vi "getAO.vi"(8 "error in (no error)":errorcluster, 11 "Instrument.LockinAPI in":refnum<class "Instrument.LockinAPI.lvclass">) -> (0 "error out":errorcluster, 2 "AOconfig":T1[](array[typedef]), 3 "Instrument.LockinAPI out":refnum<class "Instrument.LockinAPI.lvclass">)   [LabVIEW 2019, in "Instrument.LockinAPI.lvclass"]
doc: "API to get the results of lockin calculation.\n\nIf address=\"\", this API reads from localhost\nIf address is remote lockin, you need to add this computer to allowed whitelist on the lockin computer you are trying to access."
uses:
  Instrument.LockinAPI.lvclass
  C:/Users/patrick/Documents/GitHub/Instrument-Framework/lvsrc/Instrument/Instrument.lvclass
  Typedefs/LockinAPI.AOconfig--Cluster.ctl
  Typedefs/LockinAPI.Commands--Enum.ctl
  8040a651-251f-490b-970e-b747a6a9edfe.vi
  8040a651-251f-490b-970e-b747a6a9edfe.vi/73a72ad9-01cb-4234-818c-ca637e3ba3a8.vi
  8040a651-251f-490b-970e-b747a6a9edfe.vi/73a72ad9-01cb-4234-818c-ca637e3ba3a8.vi/1562ab7a-2f08-4fb7-b07f-5ee483217534.vi
  8040a651-251f-490b-970e-b747a6a9edfe.vi/73a72ad9-01cb-4234-818c-ca637e3ba3a8.vi/22dc2966-521d-4730-be92-c328b528c3eb.vi
  Instrument/Protected/Validate API method.vi
  Instrument/Private/Get RC Connection Status.vi
  Instrument/API/Send and Receive.vi
  <vilib>/Utility/Data Type/Get Type Information.vi
  <vilib>/JDP Science/JSONtext/JSON text to Variant.vi
  <vilib>/JDP Science/JSONtext/LVClass Serializer/JSONtext LVClass Serializer.lvclass
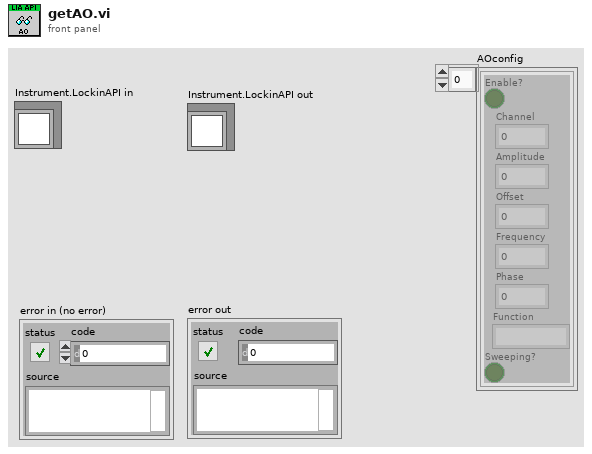
[diagram p1: front panel]
types:
  T1 = typedef "Instrument.LockinAPI.lvclass/LockinAPI.AOconfig--Cluster.ctl" = cluster{"Enable?":bool, "Channel":i32, "Amplitude":dbl, "Offset":dbl, "Frequency":dbl, "Phase":dbl, "Function":string, "Sweeping?":bool}
  T2 = typedef "Instrument.LockinAPI.lvclass/LockinAPI.Commands--Enum.ctl" = enum16{"setAI", "setAO", "setAO_Amplitude", "setAO_DC", "setAO_Frequency", "setAO_Phase", "setAO_Function", "setAO_I+", "setREF", "setREF_Frequency", "setREF_Phase", "setREF_TC", "setREF_Roll-Off", "setDAQ", "setSampling", "setOffset", "setState", "getState", "getAO", "getAI", "getResults", "getSampling", "getAOconfig", "getREFconfig", "setInputGain", "setOutputGain", "getInputGain", "getOutputGain", "setSamplingMode", "getSamplingMode", "setSweep", "setSweepTime", "setSweepTable", "getStatus", "getSweepResults", "getSweepWaveforms", "startSweep", "stopSweep", "setAUX", "getAUX"}
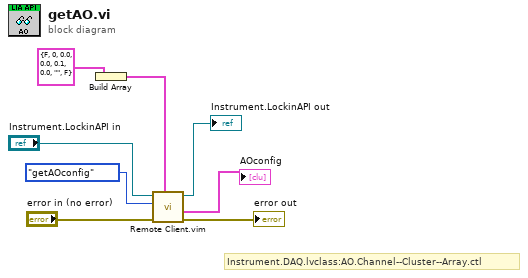
[diagram p0: block diagram]
diagram:
  # "Instrument.DAQ.lvclass:AO.Channel--Cluster--Array.ctl"
  n1 = Build Array(T1 {"Enable?"=FALSE, "Channel"=0, "Amplitude"=0.0, "Offset"=0.0, "Frequency"=0.1, "Phase"=0.0, "Function"="", "Sweeping?"=FALSE} ("AOconfig")) -> (w1:T1[])
  n2 = call "Remote Client.vim"("Data Out type"=w1, "error in (no error)"="error in (no error)", "Command in"=LockinAPI.Commands--Enum."getAOconfig" ("Command"), "Instrument in"="Instrument.LockinAPI in") -> ("error out"=→"error out":errorcluster, "Data out"=→"AOconfig":T1[], "Instrument out"=→"Instrument.LockinAPI out":refnum<class "Instrument.LockinAPI.lvclass">)  [unwired: 4 in, 1 out]
